vi "Test Debug.vi"   [LabVIEW 2019]
uses:
  <vilib>/JKI/JKI SMO/smo.lvlibp/SMO/SMO.lvclass
  Debug.lvlib
  <vilib>/addons/_JKI Toolkits/Caraya/classes/Test/Test.lvclass
  <vilib>/addons/_JKI Toolkits/Caraya/classes/Assert/Assert.lvclass
  subsystems/Attribute.Debug/DebugBehavior.ctl
  subsystems/Attribute.Debug/Attribute.Debug.lvclass
  <vilib>/addons/_JKI Toolkits/Caraya/classes/Assert/Assert Equal Value_Variant.vi
  <vilib>/addons/_JKI Toolkits/Caraya/classes/Assert/Assert Not Error.vi
types:
  T1 = typedef "Debug.lvlib/Attribute.Debug.lvclass/DebugBehavior.ctl" = enum16{"Normal", "Debug"}
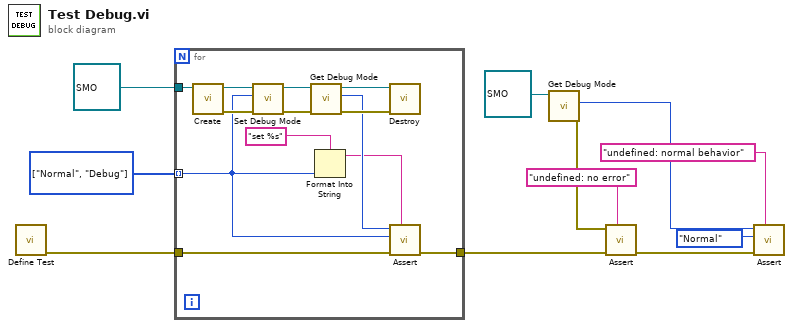
[diagram p0: block diagram]
diagram:
  w10 = T1[] [enum."Normal", enum."Debug"] items=["Normal", "Debug"] ("Array")
  n1 = call <vilib>:"Define Test.vi"() -> ("error out"=w9:errorcluster)  [unwired: 10 in, 1 out]
  n2 = for {
    tunnel: refnum<class "SMO.lvclass"> refnum ("SMO") -> [w24]
    tunnel: w10 -> [w13] mode=indexing
    tunnel: w9 -> [w17]
    tunnel: [w15] -> w6
    n3 = call <vilib>:"Create.vi"("SMO"=w24) -> ("error out"=w21:errorcluster, "SMO out"=w22:refnum<class "SMO.lvclass">)  [unwired: 8 in, 1 out]
    n4 = call "Set Debug Mode.vi"("error in (no error)"=w21, "Behavior"=w13, "SMO"=w22) -> ("error out"=w20:errorcluster, "SMO out"=w18:refnum<class "SMO.lvclass">)  [unwired: 7 in]
    n5 = call "Get Debug Mode.vi"("error in (no error)"=w20, "SMO"=w18) -> ("error out"=w19:errorcluster, "Behavior"=w16:T1, "SMO out"=w23:refnum<class "SMO.lvclass">)  [unwired: 7 in]
    n6 = Format Into String(format string="set %s", w13) -> (resulting string=w12:string)  [unwired: 2 in, 1 out]
    n7 = call <vilib>:"Destroy.vi"("error in (no error)"=w19, "SMO"=w23) -> ()  [unwired: 9 in, 1 out]
    n8 = call-poly <vilib>:"Assert.vi"("Label"=w12, "error in (no error)"=w17, "Y"=w13, "X"=w16) -> ("error out"=w15:errorcluster)  [unwired: 6 in, 1 out]
  }
  n9 = call "Get Debug Mode.vi"("SMO"=refnum<class "SMO.lvclass"> refnum) -> ("error out"=w7:errorcluster, "Behavior"=w5:T1)  [unwired: 8 in, 1 out]
  n10 = call-poly <vilib>:"Assert.vi"("Label"="undefined: no error", "error in (no error)"=w6, "Not Error?"=w7) -> ("error out"=w3:errorcluster)  [unwired: 7 in, 1 out]
  n11 = call-poly <vilib>:"Assert.vi"("Label"="undefined: normal behavior", "error in (no error)"=w3, "Y"=DebugBehavior."Normal" ("Behavior"), "X"=w5) -> ()  [unwired: 6 in, 2 out]
